vi "Module Type.vi"(11 "Sequencing in":refnum<class "Sequencing.lvclass">) -> (2 "Module Type":string)   [LabVIEW 2020, in "VolatusSeq.lvlib" / "Sequencing.lvclass"]
uses:
  Sequencing.lvclass
  Sequencing.lvclass/Sequencing.ctl
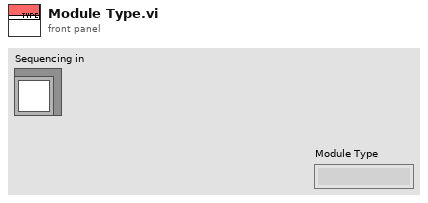
[diagram p1: front panel]
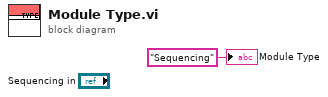
[diagram p0: block diagram]
diagram:
  "Module Type" <- "Sequencing" ("Module Type")
